vi "ConvertTextBasedCodeToLabVIEW_FixAbstractMethods.vi"(11 "String":string="   protected Subject subject;\n   public abstract void update();\n/*\n   protected Subject subject;\n   public abstract void update();\n\n*/\n   protected abstract string hello();\n//   protected abstract string hello2();") -> (3 "String 2":string)   [LabVIEW 2016]
uses:
  <vilib>/regexp/Match Regular Expression.xnode
panel:
  out "submatch 4":string
  out "whole match":string
  out "submatch 3":string
  out "submatch 2":string
  out "submatch 1":string
  out "Match":string
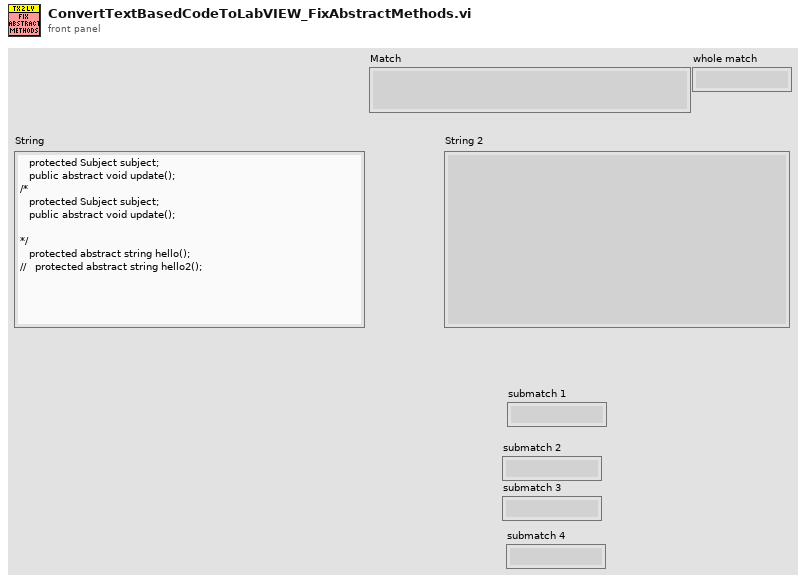
[diagram p1: front panel]
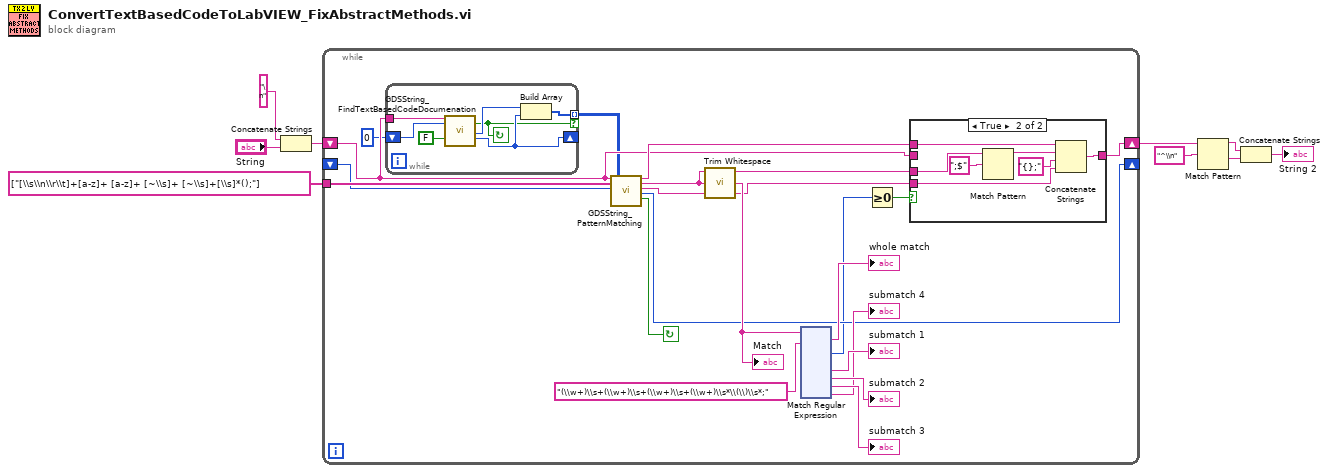
[diagram p0: block diagram]
diagram:
  n1 = Concatenate Strings("\n" ("string"), "String") -> (w6:string)
  n2 = while {
    tunnel: string[] ["[\\s\\n\\r\\t]+[a-z]+ [a-z]+ [~\\s]+ [~\\s]+[\\s]*();"] ("PatternMatchingStrings") -> [w29]
    shift-right: [w20] -> _
    shift-left: _ -> [w21]
    shift-right: [w15] -> w5
    shift-left: w6 -> [w12]
    stop <- w19 continue-if-true
    n3 = while {
      tunnel: w12 -> [w36]
      shift-right: [w34] -> _
      shift-left: 0 ("offset past match") -> [w33]
      tunnel: [w32] -> w11 mode=indexing if=w31
      stop <- w31 continue-if-true
      n4 = call <resource>:"GDSString_FindTextBasedCodeDocumenation.vi"("Text"=w36, "StringStartOffset(Default=-1 => 0 for Forward, StrLenght for Backwards)"=w33, "CommentHasToBeTheFirstItem(True)"=FALSE) -> ("Found"=w31:bool, "IndexBeforeDocument(Or after when searching Backwards)"=w35:i32, "IndexAfterDocument(Or before when searching Backwards)"=w34:i32)  [unwired: 12 in, 2 out]
      n5 = Build Array(w35, w34) -> (w32:i32[])
    }
    n6 = call <resource>:"GDSString_PatternMatching.vi"("TextIn"=w12, "PatternMatchingStrings"=w29, "StringStartOffset(Default=-1 => 0 for Forward, StrLenght for Backwards)"=w21, "IgnoreMatchesWithinThesePositions"=w11) -> ("TextBefore"=w16:string, "Match"=w14:string, "TextAfter"=w13:string, "IndexAfterMatch(Or before when searching Backwards)"=w20:i32, "Found"=w19:bool)  [unwired: 9 in, 2 out]
    n7 = call <vilib>:"Trim Whitespace.vi"("string"=w14) -> ("trimmed string"=w28:string)  [unwired: 1 in]
    "Match" <- w28
    n8 = xnode "Match Regular Expression"("input string"=w28, "regular expression"="(\\w+)\\s+(\\w+)\\s+(\\w+)\\s+(\\w+)\\s*\\(\\)\\s*;") -> ("whole match"=→"whole match":string, "offset past match"=w18:i32, "submatch 1"=→"submatch 1":string, "submatch 2"=→"submatch 2":string, "submatch 3"=→"submatch 3":string, "submatch 4"=→"submatch 4":string)  [unwired: 4 in, 3 out]
    n9 = Greater Or Equal To 0?(x=w18) -> (x >= 0?=w17:bool)
    n10 = case shown="True" w17 {
      tunnel: w16 -> [_ w39]
      tunnel: w12 -> [w37 _]
      tunnel: [w37 w40] -> w15
      tunnel: w14 -> [_ w44]
      tunnel: w13 -> [_ w38]
      frame False {
      }
      frame True {
        n11 = Match Pattern(string=w44, regular expression=";$") -> (before substring=w42:string)  [unwired: 1 in, 3 out]
        n12 = Concatenate Strings(w39, w42, "{};" ("string"), w38) -> (w40:string)
      }
    }
  }
  n13 = Match Pattern(string=w5, regular expression="^\\n") -> (before substring=w4:string, after substring=w3:string)  [unwired: 1 in, 2 out]
  n14 = Concatenate Strings(w4, w3) -> (→"String 2":string)
